vi "Test.vi"() -> ()   [LabVIEW 2014]
panel:
  out "output 2":dbl
  out "data out":string
  in  "stop":bool
  out "output 1":dbl(graph)
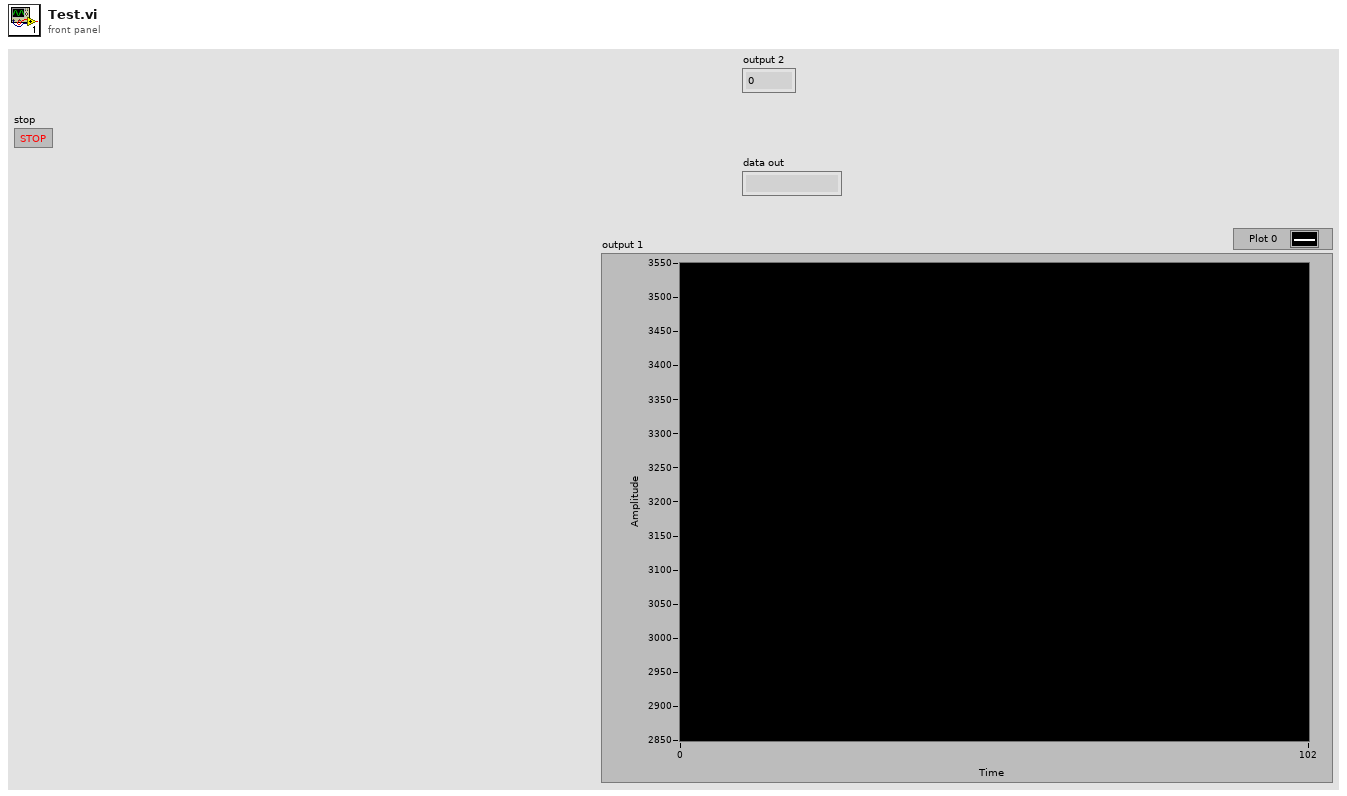
[diagram p1: front panel]
types:
  T1 = enum16{"Standard", "Buffered", "CRLF", "Immediate"}
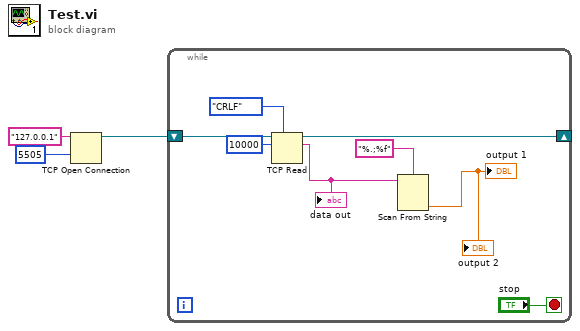
[diagram p0: block diagram]
diagram:
  n1 = TCP Open Connection(address="127.0.0.1", remote port or service name=u16 5505) -> (connection ID=w1:refnum<k5>)  [unwired: 3 in, 1 out]
  n2 = while {
    shift-right: [w8] -> _
    shift-left: w1 -> [w11]
    stop <- "stop" stop-if-true
    n3 = TCP Read(connection ID=w11, bytes to read=10000, 7:T1."CRLF" ("mode (standard)")) -> (connection ID out=w8:refnum<k5>, data out=w7:string)  [unwired: 2 in, 1 out]
    "data out" <- w7
    n4 = Scan From String(format string="%.;%f", input string=w7) -> (output 1=→"output 1" →"output 2":dbl)  [unwired: 3 in, 3 out]
  }
